vi "读取Excel文件子程序.vi"(9 "页":dbl=4.0, 10 "Filename":string) -> (1 "错误输出":errorcluster, 2 "数据":string[][](array[string]))   [LabVIEW 2013]
panel:
  out "错误输出 2":errorcluster caption="错误输出"
  in  "Excel._Application":refnum<k7>
  in  "Excel._Worksheet":refnum<k7>
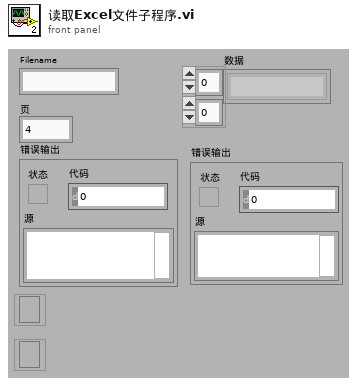
[diagram p1: front panel]
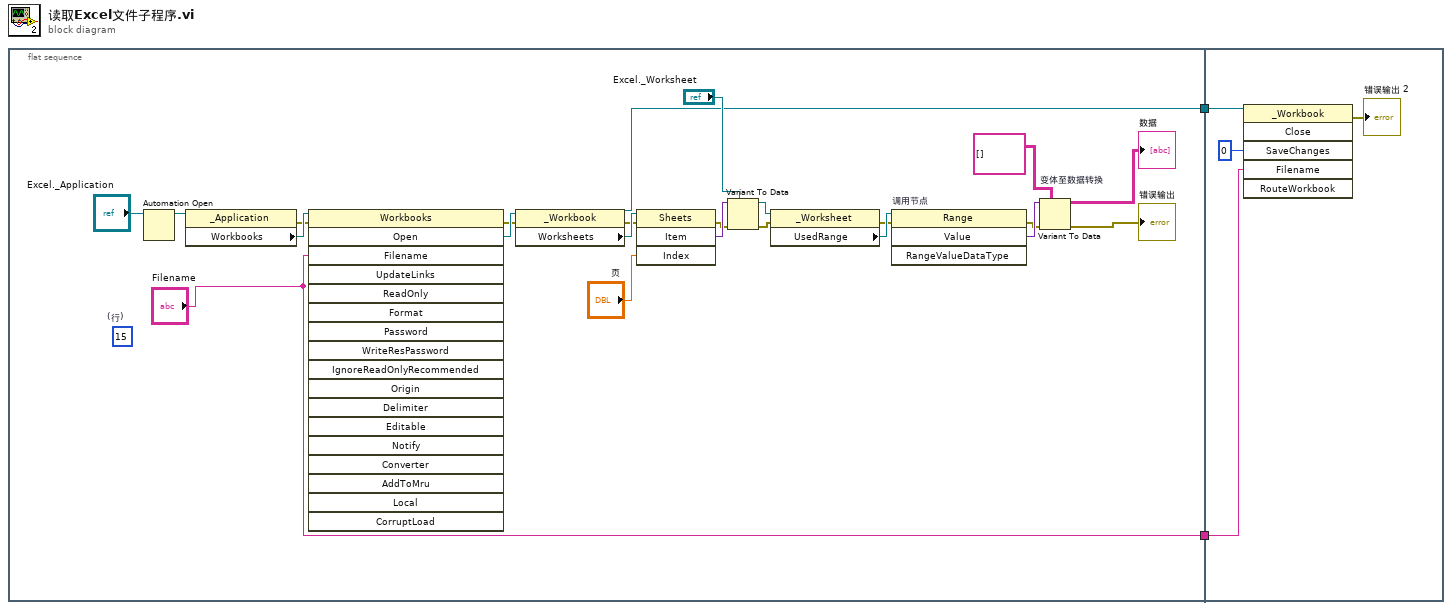
[diagram p0: block diagram]
diagram:
  n1 = flat-sequence {
    tunnel: [w5] -> w2
    tunnel: ["Filename"] -> w1
    tunnel: w2 -> [w27]
    tunnel: w1 -> [w26]
    frame #0 {
      (unwired) 15  # (行)
      n2 = Automation Open(Automation Refnum="Excel._Application") -> (Automation Refnum=w24:refnum<k7>)  [unwired: 1 in, 3 out]
      n3 = property class="_Application"(reference=w24) -> (error out=w22:errorcluster, "Workbooks"=w23:refnum<k7>)  [unwired: 1 in, 1 out]
      n4 = invoke class="Workbooks" method="Open"(reference=w23, error in=w22, "Filename"="Filename") -> (error out=w20:errorcluster, "Open"=w21:refnum<k7>)  [unwired: 15 in, 16 out]
      n5 = property class="_Workbook"(reference=w21, error in=w20) -> (reference out=w5:refnum<k7>, error out=w17:errorcluster, "Worksheets"=w18:refnum<k7>)
      n6 = invoke class="Sheets" method="Item"(reference=w18, error in=w17, "Index"="页") -> (error out=w15:errorcluster, "Item"=w16:variant)  [unwired: 1 in, 2 out]
      n7 = Variant To Data(error in=w15, type="Excel._Worksheet", Variant=w16) -> (data=w13:refnum<k7>, error out=w12:errorcluster)
      n8 = property class="_Worksheet"(reference=w13, error in=w12) -> (error out=w10:errorcluster, "UsedRange"=w11:refnum<k7>)  [unwired: 1 out]
      n9 = invoke on="调用节点" class="Range" method="Value"(reference=w11, error in=w10) -> (error out=w8:errorcluster, "Value"=w9:variant)  [unwired: 2 in, 2 out]
      n10 = Variant To Data "变体至数据转换"(error in=w8, type=string[][] [], Variant=w9) -> (data=→"数据":string[][], error out=→"错误输出":errorcluster)
    }
    frame #1 {
      n11 = invoke class="_Workbook" method="Close"(reference=w27, "SaveChanges"=0, "Filename"=w26) -> (error out=→"错误输出 2":errorcluster)  [unwired: 3 in, 5 out]
    }
  }
